vi "1D Array Variant to Key List.vi"(5 "section":string, 7 "Prefix":string, 8 "Error In":errorcluster, 11 "Variant":variant) -> (0 "Error Out":errorcluster, 2 "Key list":T1)   [LabVIEW 2015]
uses:
  <vilib>/Utility/Data Type/NI_Data Type.lvlib
panel:
  in  "Number of elements":i32
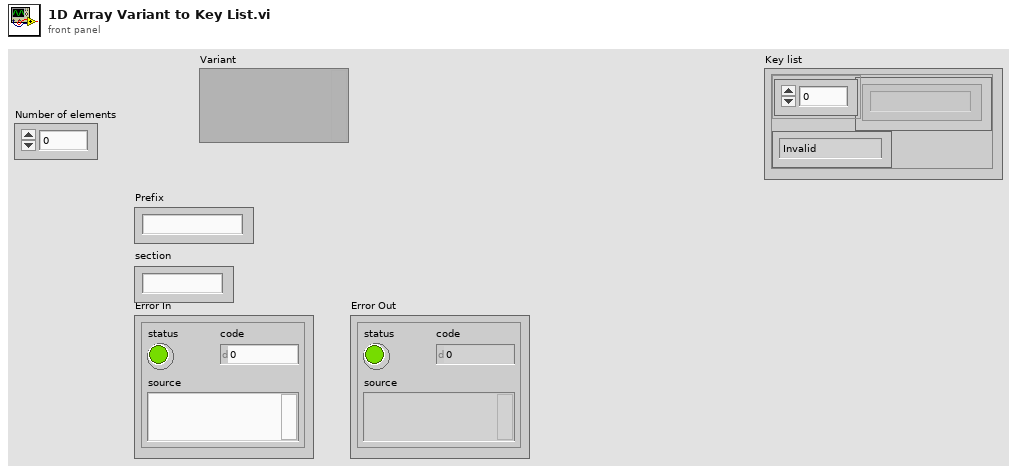
[diagram p1: front panel]
types:
  T1 = cluster{"Array":string[], "Enum":enum16{"Invalid", "Boolean", "Double", "I32", "Path", "String", "U32", "Array", "Cluster"}}
  T2 = enum16{"Invalid", "Boolean", "Double", "I32", "Path", "String", "U32", "Array", "Cluster"}
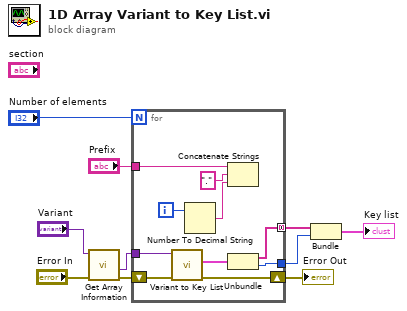
[diagram p0: block diagram]
diagram:
  n1 = call <vilib>:"Get Array Information.vi"("error in (no error)"="Error In", "Variant"="Variant") -> ("error out"=w6:errorcluster, "Array Element Data Type"=w7:variant)  [unwired: 6 in, 2 out]
  n2 = for {
    N: "Number of elements" -> [_]
    tunnel: w7 -> [w20]
    shift-right: [w18] -> w2
    shift-left: w6 -> [w19]
    tunnel: "Prefix" -> [w12]
    tunnel: [w16] -> w5 mode=concatenating
    tunnel: [w15] -> w4
    i -> [w11]
    n3 = call "Variant to Key List.vi"("Error In"=w19, "Variant"=w20) -> ("Error Out"=w18:errorcluster, "Key list"=w17:T1)  [unwired: 8 in]
    n4 = Number To Decimal String(number=w11) -> (decimal integer string=w13:string)  [unwired: 1 in]
    n5 = Concatenate Strings(w12, "." ("string"), w13) -> ()  [unwired: 1 out]
    n6 = Unbundle(w17) -> ("Array"=w16:string[], "Enum"=w15:T2)
  }
  "Error Out" <- w2
  n7 = Bundle("Array"=w5, "Enum"=w4) -> (→"Key list":T1)  [unwired: 1 in]
